vi "Receive Pattern.vi"() -> ()   [LabVIEW 2016]
panel:
  in  "Stop 2":bool
  out "Receive Fatigue":dbl(graph)
  in  "Stop":bool
  out "Received Pattern":dbl(graph)
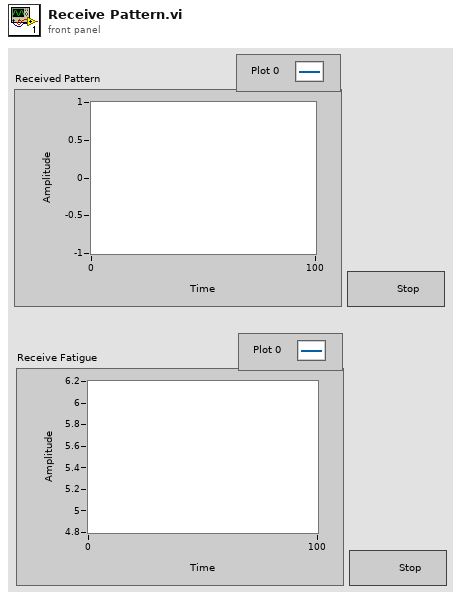
[diagram p1: front panel]
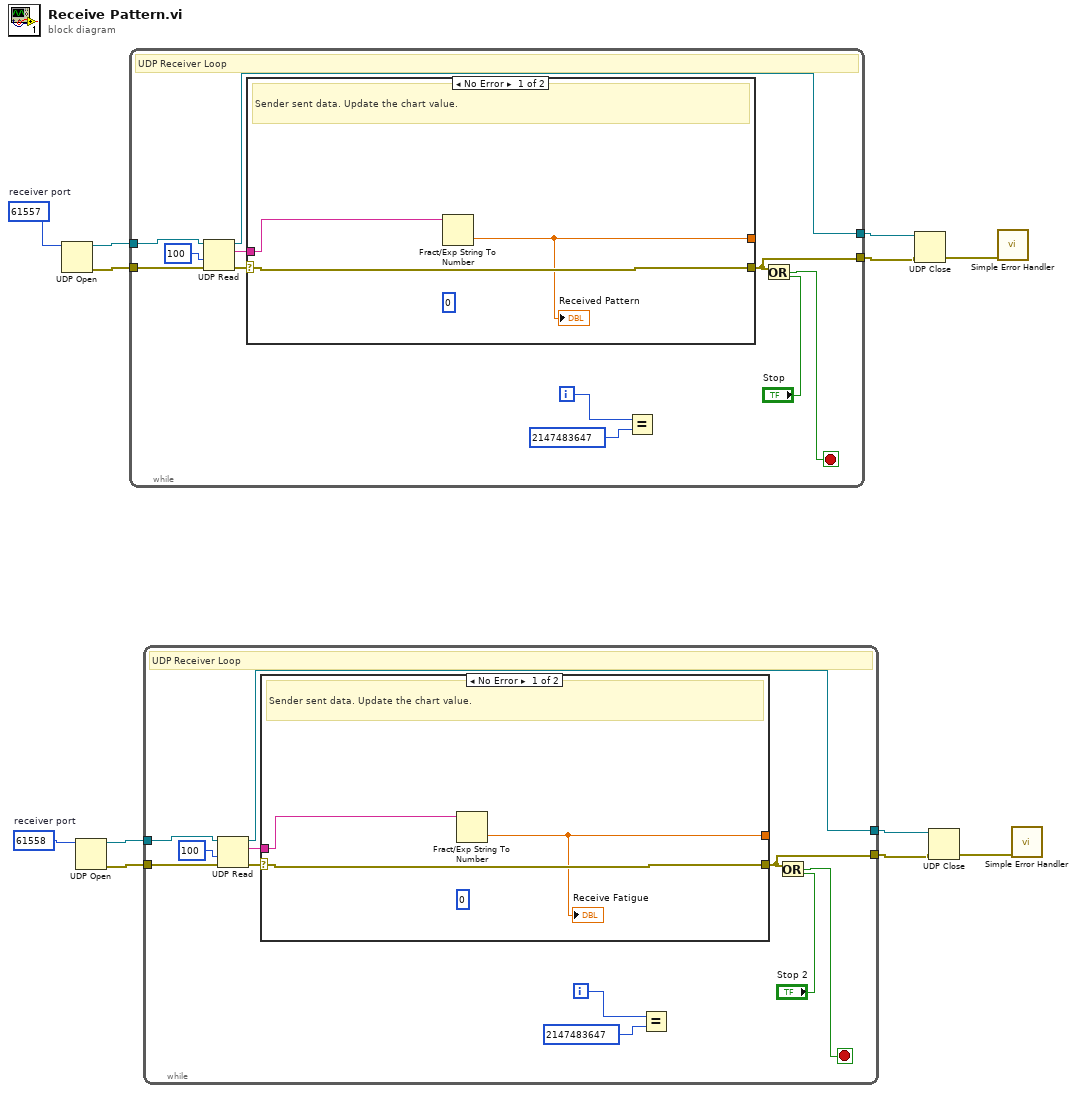
[diagram p0: block diagram]
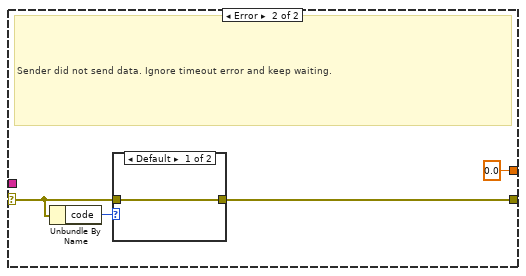
[diagram p2: hidden frame]
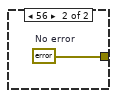
[diagram p3: hidden frame]
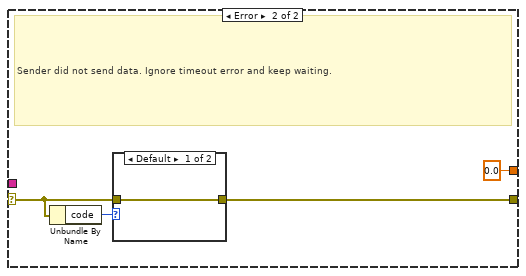
[diagram p4: hidden frame]
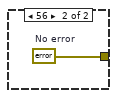
[diagram p5: hidden frame]
diagram:
  w1 = u16 61558  # receiver port
  w7 = u16 61557  # receiver port
  n1 = UDP Open(11:w7) -> (port=w8:refnum<k16>, 0:w9:errorcluster)  [unwired: 4 in, 1 out]
  n2 = UDP Open(11:w1) -> (port=w2:refnum<k16>, 0:w3:errorcluster)  [unwired: 4 in, 1 out]
  n3 = while {
    tunnel: w8 -> [w23]
    tunnel: [w16] -> w12
    tunnel: w9 -> [w21]
    tunnel: [w17] -> w10
    i -> [w15]
    stop <- w13 stop-if-true
    # "UDP Receiver Loop"
    n4 = UDP Read(connection ID=w23, timeout ms (25000)=100, 8:w21) -> (data out=w19:string, error out=w18:errorcluster, 3:w16:refnum<k16>)  [unwired: 3 out]
    n5 = case shown="No Error" w18 {
      selector: w18 -> [w26 w29]
      tunnel: w19 -> [w25 _]
      tunnel: [w26 w28] -> w17
      tunnel: [w24 0.0] -> _
      frame No Error {
        (unwired) 0 ("offset (0)")
        # "Sender sent data. Update the chart value."
        n6 = Fract/Exp String To Number(string=w25) -> (number=w24:dbl)  [unwired: 3 in, 1 out]
        "Received Pattern" <- w24
      }
      frame Error {
        # "Sender did not send data. Ignore timeout error and keep waiting."
        n7 = Unbundle By Name(w29) -> ("code"=w30:i32)
        n8 = case shown="Default" w30 {
          tunnel: w29 -> [w31 _]
          tunnel: [w31 w32] -> w28
          frame Default {
          }
          frame 56 {
            w32 = errorcluster {"status"=FALSE, "code"=0, "source"=""}  # No error
          }
        }
      }
    }
    n9 = Equal?(x=w15, y=2147483647) -> ()  [unwired: 1 out]
    n10 = Or(x=w17, y="Stop") -> (x .or. y?=w13:bool)
  }
  n11 = while {
    tunnel: w2 -> [w43]
    tunnel: [w36] -> w6
    tunnel: w3 -> [w41]
    tunnel: [w37] -> w4
    i -> [w35]
    stop <- w33 stop-if-true
    # "UDP Receiver Loop"
    n12 = UDP Read(connection ID=w43, timeout ms (25000)=100, 8:w41) -> (data out=w39:string, error out=w38:errorcluster, 3:w36:refnum<k16>)  [unwired: 3 out]
    n13 = case shown="No Error" w38 {
      selector: w38 -> [w46 w49]
      tunnel: w39 -> [w45 _]
      tunnel: [w46 w48] -> w37
      tunnel: [w44 0.0] -> _
      frame No Error {
        (unwired) 0 ("offset (0)")
        # "Sender sent data. Update the chart value."
        n14 = Fract/Exp String To Number(string=w45) -> (number=w44:dbl)  [unwired: 3 in, 1 out]
        "Receive Fatigue" <- w44
      }
      frame Error {
        # "Sender did not send data. Ignore timeout error and keep waiting."
        n15 = Unbundle By Name(w49) -> ("code"=w50:i32)
        n16 = case shown="Default" w50 {
          tunnel: w49 -> [w51 _]
          tunnel: [w51 w52] -> w48
          frame Default {
          }
          frame 56 {
            w52 = errorcluster {"status"=FALSE, "code"=0, "source"=""}  # No error
          }
        }
      }
    }
    n17 = Equal?(x=w35, y=2147483647) -> ()  [unwired: 1 out]
    n18 = Or(x=w37, y="Stop 2") -> (x .or. y?=w33:bool)
  }
  n19 = UDP Close(connection ID=w12, 8:w10) -> (error out=w11:errorcluster)  [unwired: 1 out]
  n20 = UDP Close(connection ID=w6, 8:w4) -> (error out=w5:errorcluster)  [unwired: 1 out]
  n21 = call <vilib>:"Simple Error Handler.vi"("error in (no error)"=w11) -> ()  [unwired: 1 in, 8 out]
  n22 = call <vilib>:"Simple Error Handler.vi"("error in (no error)"=w5) -> ()  [unwired: 1 in, 8 out]
